vi "Write Report.vi"(10 "Data":string[][](array[string]), 11 "file path":path caption="文件路径 （空时为对话框）") -> ()   [LabVIEW 2014]
uses:
  <vilib>/Utility/file.llb/Write To Spreadsheet File (string).vi
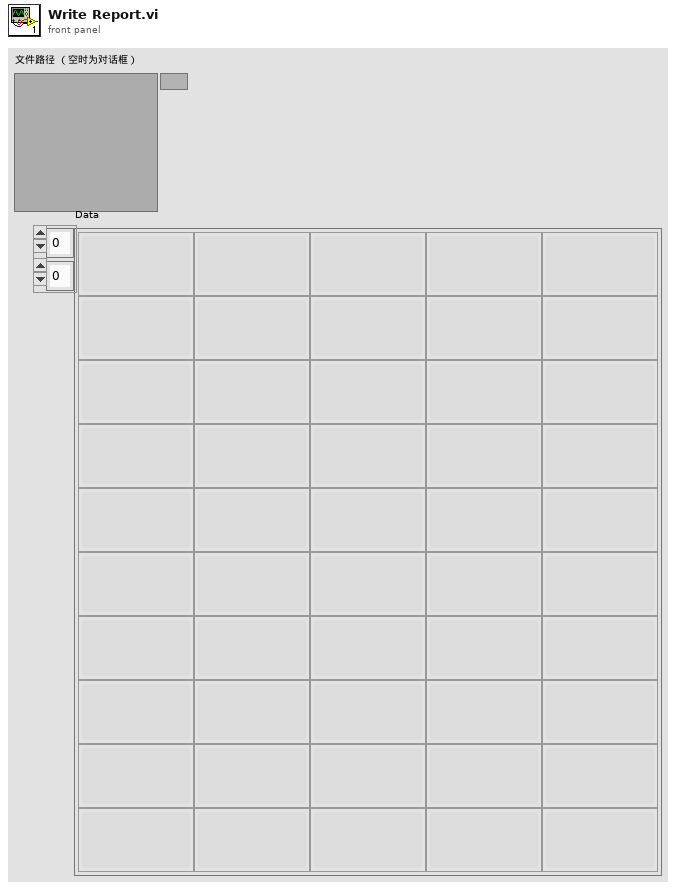
[diagram p1: front panel]
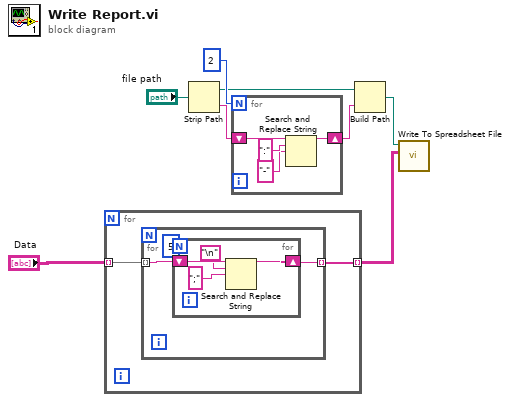
[diagram p0: block diagram]
diagram:
  n1 = for {
    tunnel: [w10] -> w2 mode=indexing
    tunnel: "Data" -> [w9] mode=indexing
    n2 = for {
      tunnel: [w12] -> w10 mode=indexing
      tunnel: w9 -> [w13] mode=indexing
      n3 = for {
        N: 5 -> [_]
        shift-right: [w15] -> w12
        shift-left: w13 -> [w16]
        n4 = Search and Replace String(input string=w16, search string="\n", replace string=";" ("替换字符串(\"\")")) -> (result string=w15:string)  [unwired: 5 in, 3 out]
      }
    }
  }
  n5 = Strip Path(path="file path") -> (stripped path=w5:path, name=w6:string)
  n6 = for {
    N: 2 -> [_]
    shift-right: [w18] -> w4
    shift-left: w6 -> [w21]
    n7 = Search and Replace String(input string=w21, search string=":" ("搜索字符串"), replace string="-" ("替换字符串(\"\")")) -> (result string=w18:string)  [unwired: 5 in, 3 out]
  }
  n8 = Build Path(base path=w5, name or relative path=w4) -> (appended path=w3:path)
  n9 = call-poly <vilib>:"Write To Spreadsheet File.vi"("2D data"=w2, "file path (dialog if empty)"=w3) -> ()  [unwired: 6 in, 1 out]
